vi "_Create.vi"(8 "error in (no error)":errorcluster, 9 "Data":string, 10 "ID":string, 11 "Message in":refnum<class "Message.lvclass">) -> (0 "error out":errorcluster, 3 "Message out":refnum<class "Message.lvclass">)   [LabVIEW 2020, in "Stream-Simple-Msg.lvlib" / "Message.lvclass"]
uses:
  Message.lvclass
  Message.lvclass/Message.ctl
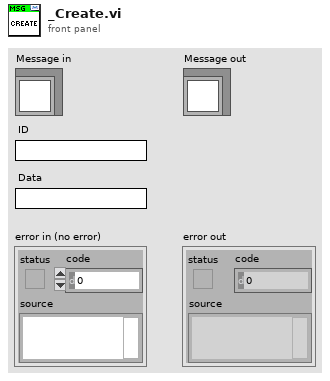
[diagram p1: front panel]
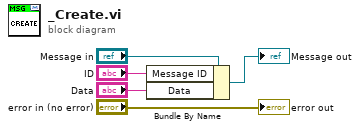
[diagram p0: block diagram]
diagram:
  n1 = Bundle By Name(cluster="Message in", "Message ID"="ID", "Data"="Data") -> (→"Message out":refnum<class "Message.lvclass">)
  "error out" <- "error in (no error)"
